vi "Load_v5.vi"(8 "error in":errorcluster, 11 "Path (open dialog)":path) -> (0 "error out":errorcluster, 1 "cancelled":bool, 2 "Procedure Name":string, 3 "Chosen Path":path, 4 "Save Cluster":T1={"Version"="", "Devices"=[], "Select Layout"=0, "Layout:Strings And Values []"=[], "User defined functions"="-- -------------------------------------------------------------------------------------------\n-- The following functions are part of the \"standard load\" of functions and should not be messed with\n-- They are here for reference only.\n-- Please add any user functions above this comment\n-- -------------------------------------------------------------------------------------------\n\n-- Creates a linear ramp from A to B\nfunction LineRamp(f, Initial, Final)\n    return (1-f)*Initial + f*Final;\nend\n\n-- Creates an exponential ramp from A to B\nfunction ExpRamp(t, a, b, tau)\n   return (b - a*exp(tMax / tau) + (a-b)*exp(t/tau))/ ( 1 - exp(tMax / tau) );\nend\n\n-- Creates a sinewave\nfunction SinRamp(t,Offset,A,Freq, Phase)\n    return Offset + A * sin(2*pi*Freq*t + Phase)\nend\n\n-- Creates a blackman pulse\nfunction Blackman(f, Offset, A)\n    return Offset +  A*sqrt(0.5*cos(3.1415*(2*f-1))+0.08*cos(2*pi*(2*f-1))+0.42);\nend\n\n-- Creates a half-gauss ramp\nfunction HalfGaussRamp(t, a, b, Width)\n    local y;\n    y = exp(-(tMax^2)/Width^2);\n    y = (a -  b*y)/(1-y)  +  ((b-a)/(1-y))*exp(-((t-tMax)^2)/Width^2);\n    return y;\nend\n\n-- Creates an \"O'Hara\" ramp from A to B, for dipole evaporation\nfunction EvapRamp(t, a, b, tau)\n   local y;\n  y = log(a/b) / log(1+tMax/tau);\n  y = a * (1+t/tau)^(-y);\n  return y;\nend\n", "VariableManager"=refnum} {"Select Layout" items=["Default"]})   [LabVIEW 2013]
doc: "Load entire SetList configuration to disk. This includes Device configuration, software image, user procedures, variables, layouts.\n\nIf no \"path\" to file is given, the user is presented with a dialog box. The chosen full path is returned, as well as the file name as \"Procedure Name.\""
uses:
  TypeDefs/SaveCluster.ctl
  VariableManagerCodes/VariableManager/VariableManager.lvclass
  DeviceVIs/Device/Device.lvclass
  <vilib>/Utility/miscctls.llb/LVStringsAndValuesArrayTypeDef_I32.ctl
panel:
  # "note: if user cancels, will also throw an\nerror (code 43)"
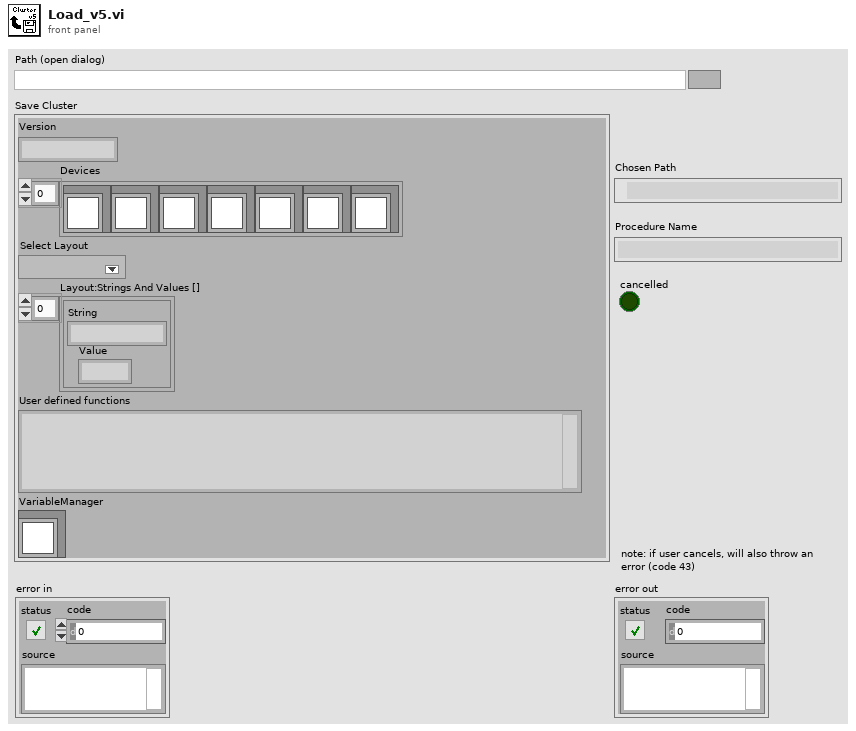
[diagram p1: front panel]
types:
  T1 = typedef "SaveCluster.ctl" = cluster{"Version":string, "Devices":refnum<class "Device.lvclass">[], "Select Layout":i32, "Layout:Strings And Values []":T2, "User defined functions":string, "VariableManager":refnum<class "VariableManager.lvclass">}
  T2 = typedef "LVStringsAndValuesArrayTypeDef_I32.ctl" = cluster{"String":string, "Value":i32}[]
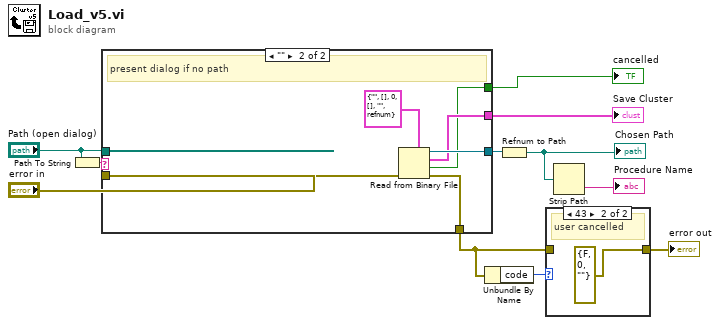
[diagram p0: block diagram]
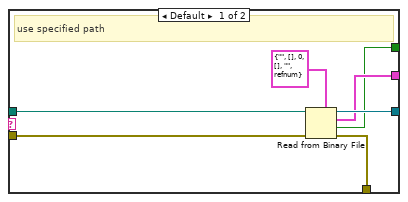
[diagram p3: hidden frame]
diagram:
  n1 = Path To String(path="Path (open dialog)") -> (string=w3:string)
  n2 = case shown="\"\"" w3 {
    tunnel: [w15 w22] -> w11
    tunnel: [w18 w24] -> w7
    tunnel: "Path (open dialog)" -> [w17 _]
    tunnel: "error in" -> [w16 w23]
    tunnel: [w14 w21] -> w5
    tunnel: [w12 w19] -> w1
    frame Default {
      # "use specified path"
      n3 = Read from Binary File(5:T1 {"Version"="", "Devices"=[], "Select Layout"=0, "Layout:Strings And Values []"=[], "User defined functions"="", "VariableManager"=refnum} ("Save Cluster"), 8:w16, 11:w17) -> (0:w18:errorcluster, 1:w12:bool, 2:w14:T1, 3:w15:refnum<file>)  [unwired: 3 in]
    }
    frame "" {
      # "present dialog if no path"
      n4 = Read from Binary File(5:T1 {"Version"="", "Devices"=[], "Select Layout"=0, "Layout:Strings And Values []"=[], "User defined functions"="", "VariableManager"=refnum} ("Save Cluster"), 8:w23) -> (0:w24:errorcluster, 1:w19:bool, 2:w21:T1, 3:w22:refnum<file>)  [unwired: 4 in]
    }
  }
  "Save Cluster" <- w5
  "cancelled" <- w1
  n5 = Unbundle By Name(w7) -> ("code"=w8:i32)
  n6 = Refnum to Path(1:w11) -> (0:w10:path)
  "Chosen Path" <- w10
  n7 = case shown="43" w8 {
    tunnel: w7 -> [w25 _]
    tunnel: [w25 errorcluster {"status"=FALSE, "code"=0, "source"=""} ("error out")] -> w6
    frame Default {
      # "pass other"
    }
    frame 43 {
      # "user cancelled"
    }
  }
  "error out" <- w6
  n8 = Strip Path(path=w10) -> (name=→"Procedure Name":string)  [unwired: 1 out]
